vi "Motic Set Bit Count.vi"(8 "error in (no error)":errorcluster, 10 "bit":i32, 11 "camera":i32) -> (0 "error out":errorcluster, 3 "camera out":i32)   [LabVIEW 2012, in "MoticApi.lvlib"]
doc: "MOTICAPI bool Motic_setBitCount(MUCam_Handle camera, int bit);"
uses:
  MoticApi.lvlib
  MoticApi.dll
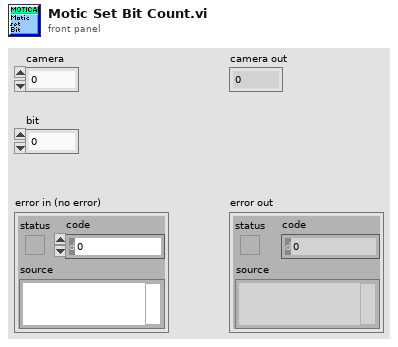
[diagram p1: front panel]
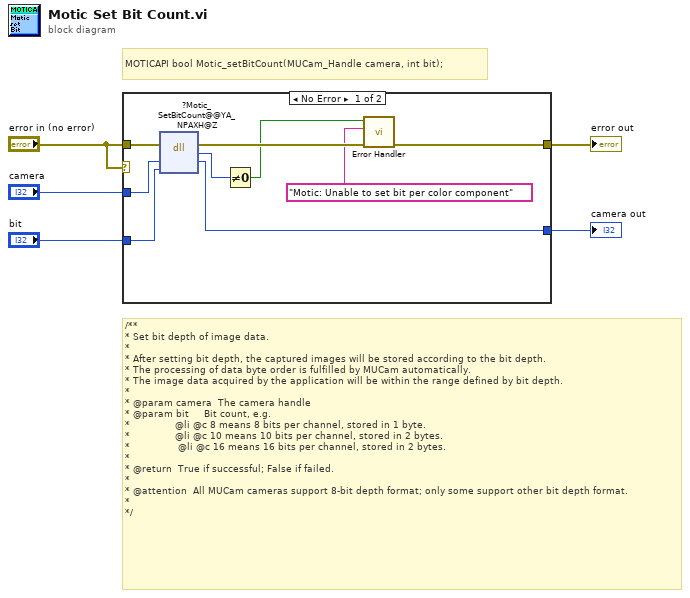
[diagram p0: block diagram]
diagram:
  # "/**\n* Set bit depth of image data.\n*\n* After setting bit depth, the captured images will be stored according to the bit depth.\n* The processing of data byte order is fulfilled by MUCam automatically.\n* The image data acquired by the application will be within the range defined by bit depth.\n*\n* @param camera  The camera handle\n* @param bit     Bit count, e.g.\n*\t              @li @c 8 means 8 bits per channel, stored in 1 byte.\n*\t              @li @c 10 means 10 bits per channel, stored in 2 bytes.\n*                @li @c 16 means 16 bits per channel, stored in 2 bytes.\n*\n* @return  True if successful; False if failed.\n*\n* @attention  All MUCam cameras support 8-bit depth format; only some support other bit depth format.\n*\n*/"
  # "MOTICAPI bool Motic_setBitCount(MUCam_Handle camera, int bit);"
  n1 = case shown="No Error" "error in (no error)" {
    tunnel: "camera" -> [w13 w15]
    tunnel: [w12 w15] -> w4
    tunnel: "bit" -> [w11 _]
    tunnel: "error in (no error)" -> [w10 w16]
    tunnel: [w8 w16] -> w2
    frame No Error {
      n2 = dll-call lib="C:/Users/TTS-Digital/Desktop/MoticApi/MoticApi_git/MoticApi/MoticApi.*" fn="?Motic_SetBitCount@@YA_NPAXH@Z"(error in=w10, "camera"=w13, "bit"=w11) -> (error out=w9:errorcluster, "return type"=w14:u8, "camera"=w12:i32)  [unwired: 3 in, 1 out]
      n3 = Not Equal To 0?(x=w14) -> (x != 0?=w7:bool)
      n4 = call "Error Handler.vi"("error in (no error)"=w9, "Error message"="Motic: Unable to set bit per color component" ("error message (\"\")"), "Function return"=w7) -> ("error out"=w8:errorcluster)  [unwired: 8 in]
    }
    frame Error {
    }
  }
  "camera out" <- w4
  "error out" <- w2
